vi "setStages.vi"(8 "error in (no error)":errorcluster, 10 "Stage":string, 11 "RampEvent.lvclass in":refnum<class "RampEvent.lvclass">) -> (0 "error out":errorcluster, 3 "RampEvent.lvclass out":refnum<class "RampEvent.lvclass">)   [LabVIEW 2011, in "Tools.lvlib" / "Scripting.lvlib" / "RampEvent.lvclass"]
uses:
  RampEvent.lvclass
  ScriptEvent.lvclass
  RampEvent.lvclass/RampEvent.ctl
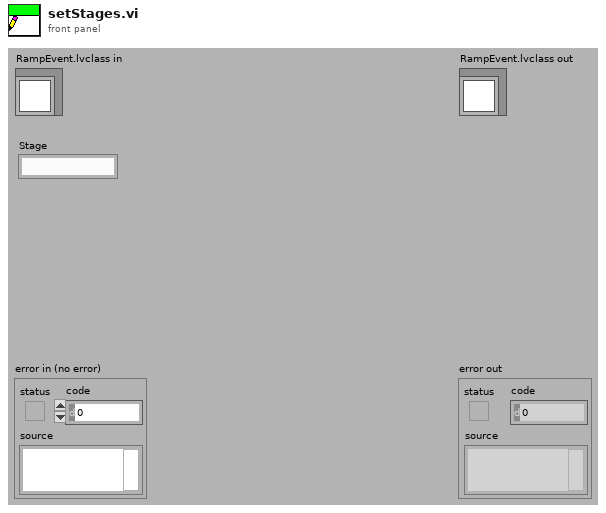
[diagram p1: front panel]
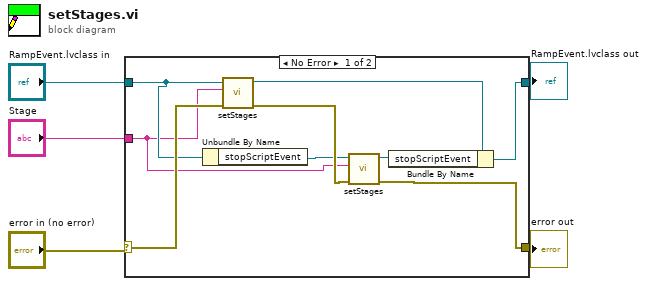
[diagram p0: block diagram]
diagram:
  n1 = case shown="No Error" "error in (no error)" {
    selector: "error in (no error)" -> [w14 w15]
    tunnel: [w10 w15] -> w4
    tunnel: "RampEvent.lvclass in" -> [w13 w16]
    tunnel: [w11 w16] -> w2
    tunnel: "Stage" -> [w6 _]
    frame No Error {
      n2 = Unbundle By Name(w13) -> ("stopScriptEvent"=w8:refnum<class "ScriptEvent.lvclass">)
      n3 = call-parent "setStages.vi"("error in (no error)"=w14, "Stage"=w6, "ScriptEvent.lvclass in"=w13) -> ("error out"=w9:errorcluster, "ScriptEvent.lvclass out"=w12:refnum<class "RampEvent.lvclass">)  [unwired: 7 in]
      n4 = call-dynamic "setStages.vi"("error in (no error)"=w9, "Stage"=w6, "ScriptEvent.lvclass in"=w8) -> ("error out"=w10:errorcluster, "ScriptEvent.lvclass out"=w7:refnum<class "ScriptEvent.lvclass">)  [unwired: 7 in]
      n5 = Bundle By Name(cluster=w12, "stopScriptEvent"=w7) -> (w11:refnum<class "RampEvent.lvclass">)
    }
    frame Error {
    }
  }
  "error out" <- w4
  "RampEvent.lvclass out" <- w2
